vi "FaulhaberV3-Ascii_V1.vi"() -> (1 "searchnames":string[](array[string]), 2 "ID":u32[](array[numeric]), 3 "Faulhaber Objects":T3(array[cluster]))   [LabVIEW 2011] (continued)
\t<CANopenSubObject subIndex=\"0E\" name=\"Motor NTC offset\" objectType=\"7\" dataType=\"0003\" lowLimit=\"0xFFFF8000\" accessType=\"ro\" PDOmapping=\"no\" objFlags=\"00030000\" />\n\t\t\t\t\t</CANopenObject>\n\t\t\t\t\t<CANopenObject index=\"2501\" name=\"Hall scaling\" objectType=\"9\" subNumber=\"15\">\n\t\t\t\t\t\t<CANopenSubObject subIndex=\"00\" name=\"Number of entries\" objectType=\"7\" dataType=\"0005\" accessType=\"ro\" defaultValue=\"14\" PDOmapping=\"no\" />\n\t\t\t\t\t\t<CANopenSubObject subIndex=\"01\" name=\"Gain A\" objectType=\"7\" dataType=\"0006\" accessType=\"ro\" PDOmapping=\"no\" objFlags=\"00030000\" />\n\t\t\t\t\t\t<CANopenSubObject subIndex=\"02\" name=\"Hall A  offset\" objectType=\"7\" dataType=\"0006\" accessType=\"ro\" PDOmapping=\"no\" objFlags=\"00030000\" />\n\t\t\t\t\t\t<CANopenSubObject subIndex=\"03\" name=\"Hall A sin\" objectType=\"7\" dataType=\"0006\" accessType=\"ro\" PDOmapping=\"no\" objFlags=\"00030000\" />\n\t\t\t\t\t\t<CANopenSubObject subIndex=\"04\" name=\"Hall A cos\" objectType=\"7\" dataType=\"0006\" accessType=\"ro\" PDOmapping=\"no\" objFlags=\"00030000\" />\n\t\t\t\t\t\t<CANopenSubObject subIndex=\"05\" name=\"Corr A\" objectType=\"7\" dataType=\"0006\" accessType=\"ro\" PDOmapping=\"no\" objFlags=\"00030000\" />\n\t\t\t\t\t\t<CANopenSubObject subIndex=\"06\" name=\"Hall B offset\" objectType=\"7\" dataType=\"0006\" accessType=\"ro\" PDOmapping=\"no\" objFlags=\"00030000\" />\n\t\t\t\t\t\t<CANopenSubObject subIndex=\"07\" name=\"Hall B sin\" objectType=\"7\" dataType=\"0006\" accessType=\"ro\" PDOmapping=\"no\" objFlags=\"00030000\" />\n\t\t\t\t\t\t<CANopenSubObject subIndex=\"08\" name=\"Hall B cos\" objectType=\"7\" dataType=\"0006\" accessType=\"ro\" PDOmapping=\"no\" objFlags=\"00030000\" />\n\t\t\t\t\t\t<CANopenSubObject subIndex=\"09\" name=\"Corr B\" objectType=\"7\" dataType=\"0006\" accessType=\"ro\" PDOmapping=\"no\" objFlags=\"00030000\" />\n\t\t\t\t\t\t<CANopenSubObject subIndex=\"0A\" name=\"Hall C offset\" objectType=\"7\" dataType=\"0006\" accessType=\"ro\" PDOmapping=\"no\" objFlags=\"00030000\" />\n\t\t\t\t\t\t<CANopenSubObject subIndex=\"0B\" name=\"Hall C sin\" objectType=\"7\" dataType=\"0006\" accessType=\"ro\" PDOmapping=\"no\" objFlags=\"00030000\" />\n\t\t\t\t\t\t<CANopenSubObject subIndex=\"0C\" name=\"Hall C cos\" objectType=\"7\" dataType=\"0006\" accessType=\"ro\" PDOmapping=\"no\" objFlags=\"00030000\" />\n\t\t\t\t\t\t<CANopenSubObject subIndex=\"0D\" name=\"Offset A\" objectType=\"7\" dataType=\"0006\" accessType=\"ro\" PDOmapping=\"no\" objFlags=\"00030000\" />\n\t\t\t\t\t\t<CANopenSubObject subIndex=\"0E\" name=\"Offset B\" objectType=\"7\" dataType=\"0006\" accessType=\"ro\" PDOmapping=\"no\" objFlags=\"00030000\" />\n\t\t\t\t\t</CANopenObject>\n\t\t\t\t\t<CANopenObject index=\"2502\" name=\"Internal filter parameters\" objectType=\"9\" subNumber=\"14\">\n\t\t\t\t\t\t<CANopenSubObject subIndex=\"00\" name=\"Number of entries\" objectType=\"7\" dataType=\"0005\" accessType=\"ro\" defaultValue=\"13\" PDOmapping=\"no\" />\n\t\t\t\t\t\t<CANopenSubObject subIndex=\"01\" name=\"Filter time actual velocity\" objectType=\"7\" dataType=\"0006\" lowLimit=\"0\" highLimit=\"65535\" accessType=\"rw\" defaultValue=\"256\" PDOmapping=\"no\" objFlags=\"00020000\" />\n\t\t\t\t\t\t<CANopenSubObject subIndex=\"02\" name=\"Filter time IA \" objectType=\"7\" dataType=\"0006\" accessType=\"ro\" PDOmapping=\"no\" objFlags=\"00030000\" />\n\t\t\t\t\t\t<CANopenSubObject subIndex=\"03\" name=\"Filter time IB\" objectType=\"7\" dataType=\"0006\" accessType=\"ro\" PDOmapping=\"no\" objFlags=\"00030000\" />\n\t\t\t\t\t\t<CANopenSubObject subIndex=\"04\" name=\"Filter time IC\" objectType=\"7\" dataType=\"0006\" accessType=\"ro\" PDOmapping=\"no\" objFlags=\"00030000\" />\n\t\t\t\t\t\t<CANopenSubObject subIndex=\"05\" name=\"Filter time Uel\" objectType=\"7\" dataType=\"0006\" accessType=\"ro\" PDOmapping=\"no\" objFlags=\"00030000\" />\n\t\t\t\t\t\t<CANopenSubObject subIndex=\"06\" name=\"Filter time Umot\" objectType=\"7\" dataType=\"0006\" accessType=\"ro\" PDOmapping=\"no\" objFlags=\"00030000\" />\n\t\t\t\t\t\t<CANopenSubObject subIndex=\"07\" name=\"Additional filter time Uel\" objectType=\"7\" dataType=\"0006\" lowLimit=\"0x0\" accessType=\"ro\" PDOmapping=\"no\" objFlags=\"00030000\" />\n\t\t\t\t\t\t<CANopenSubObject subIndex=\"08\" name=\"Additional filter time Umot\" objectType=\"7\" dataType=\"0006\" lowLimit=\"0x0\" accessType=\"ro\" PDOmapping=\"no\" objFlags=\"00030000\" />\n\t\t\t\t\t\t<CANopenSubObject subIndex=\"09\" name=\"Filter time Iq thermal model\" objectType=\"7\" dataType=\"0006\" accessType=\"ro\" PDOmapping=\"no\" objFlags=\"00030000\" />\n\t\t\t\t\t\t<CANopenSubObject subIndex=\"0A\" name=\"Filter time Id thermal model\" objectType=\"7\" dataType=\"0006\" accessType=\"ro\" PDOmapping=\"no\" objFlags=\"00030000\" />\n\t\t\t\t\t\t<CANopenSubObject subIndex=\"0B\" name=\"Filter time Imot thermal model\" objectType=\"7\" dataType=\"0006\" accessType=\"ro\" PDOmapping=\"no\" objFlags=\"00030000\" />\n\t\t\t\t\t\t<CANopenSubObject subIndex=\"0C\" name=\"Filter time setpoint voltage model\" objectType=\"7\" dataType=\"0006\" accessType=\"ro\" PDOmapping=\"no\" objFlags=\"00030000\" />\n\t\t\t\t\t\t<CANopenSubObject subIndex=\"0D\" name=\"Filter time electrical time constant\" objectType=\"7\" dataType=\"0006\" lowLimit=\"0\" highLimit=\"65535\" accessType=\"rw\" PDOmapping=\"no\" objFlags=\"00020000\" />\n\t\t\t\t\t</CANopenObject>\n\t\t\t\t\t<CANopenObject index=\"2503\" name=\"Boot options\" objectType=\"7\" dataType=\"0006\" lowLimit=\"0\" highLimit=\"2\" accessType=\"rw\" defaultValue=\"1\" PDOmapping=\"no\" objFlags=\"00020000\" />\n\t\t\t\t\t<CANopenObject index=\"2504\" name=\"Hall compensation\" objectType=\"9\" subNumber=\"13\">\n\t\t\t\t\t\t<CANopenSubObject subIndex=\"00\" name=\"Number of entries\" objectType=\"7\" dataType=\"0005\" accessType=\"ro\" defaultValue=\"12\" PDOmapping=\"no\" />\n\t\t\t\t\t\t<CANopenSubObject subIndex=\"01\" name=\"Entry 01\" objectType=\"7\" dataType=\"0003\" accessType=\"ro\" PDOmapping=\"no\" objFlags=\"00030000\" />\n\t\t\t\t\t\t<CANopenSubObject subIndex=\"02\" name=\"Entry 02\" objectType=\"7\" dataType=\"0003\" accessType=\"ro\" PDOmapping=\"no\" objFlags=\"00030000\" />\n\t\t\t\t\t\t<CANopenSubObject subIndex=\"03\" name=\"Entry 03\" objectType=\"7\" dataType=\"0003\" accessType=\"ro\" PDOmapping=\"no\" objFlags=\"00030000\" />\n\t\t\t\t\t\t<CANopenSubObject subIndex=\"04\" name=\"Entry 04\" objectType=\"7\" dataType=\"0003\" accessType=\"ro\" PDOmapping=\"no\" objFlags=\"00030000\" />\n\t\t\t\t\t\t<CANopenSubObject subIndex=\"05\" name=\"Entry 05\" objectType=\"7\" dataType=\"0003\" accessType=\"ro\" PDOmapping=\"no\" objFlags=\"00030000\" />\n\t\t\t\t\t\t<CANopenSubObject subIndex=\"06\" name=\"Entry 06\" objectType=\"7\" dataType=\"0003\" accessType=\"ro\" PDOmapping=\"no\" objFlags=\"00030000\" />\n\t\t\t\t\t\t<CANopenSubObject subIndex=\"07\" name=\"Entry 07\" objectType=\"7\" dataType=\"0003\" accessType=\"ro\" PDOmapping=\"no\" objFlags=\"00030000\" />\n\t\t\t\t\t\t<CANopenSubObject subIndex=\"08\" name=\"Entry 08\" objectType=\"7\" dataType=\"0003\" accessType=\"ro\" PDOmapping=\"no\" objFlags=\"00030000\" />\n\t\t\t\t\t\t<CANopenSubObject subIndex=\"09\" name=\"Entry 09\" objectType=\"7\" dataType=\"0003\" accessType=\"ro\" PDOmapping=\"no\" objFlags=\"00030000\" />\n\t\t\t\t\t\t<CANopenSubObject subIndex=\"0A\" name=\"Entry 10\" objectType=\"7\" dataType=\"0003\" accessType=\"ro\" PDOmapping=\"no\" objFlags=\"00030000\" />\n\t\t\t\t\t\t<CANopenSubObject subIndex=\"0B\" name=\"Entry 11\" objectType=\"7\" dataType=\"0003\" accessType=\"ro\" PDOmapping=\"no\" objFlags=\"00030000\" />\n\t\t\t\t\t\t<CANopenSubObject subIndex=\"0C\" name=\"Entry 12\" objectType=\"7\" dataType=\"0003\" accessType=\"ro\" PDOmapping=\"no\" objFlags=\"00030000\" />\n\t\t\t\t\t</CANopenObject>\n\t\t\t\t\t<CANopenObject index=\"2506\" name=\"Encoder compensation\" objectType=\"9\" subNumber=\"65\">\n\t\t\t\t\t\t<CANopenSubObject subIndex=\"00\" name=\"Number of entries\" objectType=\"7\" dataType=\"0005\" accessType=\"ro\" defaultValue=\"64\" PDOmapping=\"no\" />\n\t\t\t\t\t\t<CANopenSubObject subIndex=\"01\" name=\"Value 0\" objectType=\"7\" dataType=\"0003\" lowLimit=\"-32768\" highLimit=\"32767\" accessType=\"rw\" defaultValue=\"0\" PDOmapping=\"no\" objFlags=\"00020000\" />\n\t\t\t\t\t\t<CANopenSubObject subIndex=\"02\" name=\"Value 1\" objectType=\"7\" dataType=\"0003\" lowLimit=\"-32768\" highLimit=\"32767\" accessType=\"rw\" defaultValue=\"0\" PDOmapping=\"no\" objFlags=\"00020000\" />\n\t\t\t\t\t\t<CANopenSubObject subIndex=\"03\" name=\"Value 2\" objectType=\"7\" dataType=\"0003\" lowLimit=\"-32768\" highLimit=\"32767\" accessType=\"rw\" defaultValue=\"0\" PDOmapping=\"no\" objFlags=\"00020000\" />\n\t\t\t\t\t\t<CANopenSubObject subIndex=\"04\" name=\"Value 3\" objectType=\"7\" dataType=\"0003\" lowLimit=\"-32768\" highLimit=\"32767\" accessType=\"rw\" defaultValue=\"0\" PDOmapping=\"no\" objFlags=\"00020000\" />\n\t\t\t\t\t\t<CANopenSubObject subIndex=\"05\" name=\"Value 4\" objectType=\"7\" dataType=\"0003\" lowLimit=\"-32768\" highLimit=\"32767\" accessType=\"rw\" defaultValue=\"0\" PDOmapping=\"no\" objFlags=\"00020000\" />\n\t\t\t\t\t\t<CANopenSubObject subIndex=\"06\" name=\"Value 5\" objectType=\"7\" dataType=\"0003\" lowLimit=\"-32768\" highLimit=\"32767\" accessType=\"rw\" defaultValue=\"0\" PDOmapping=\"no\" objFlags=\"00020000\" />\n\t\t\t\t\t\t<CANopenSubObject subIndex=\"07\" name=\"Value 6\" objectType=\"7\" dataType=\"0003\" lowLimit=\"-32768\" highLimit=\"32767\" accessType=\"rw\" defaultValue=\"0\" PDOmapping=\"no\" objFlags=\"00020000\" />\n\t\t\t\t\t\t<CANopenSubObject subIndex=\"08\" name=\"Value 7\" objectType=\"7\" dataType=\"0003\" lowLimit=\"-32768\" highLimit=\"32767\" accessType=\"rw\" defaultValue=\"0\" PDOmapping=\"no\" objFlags=\"00020000\" />\n\t\t\t\t\t\t<CANopenSubObject subIndex=\"09\" name=\"Value 8\" objectType=\"7\" dataType=\"0003\" lowLimit=\"-32768\" highLimit=\"32767\" accessType=\"rw\" defaultValue=\"0\" PDOmapping=\"no\" objFlags=\"00020000\" />\n\t\t\t\t\t\t<CANopenSubObject subIndex=\"0A\" name=\"Value 9\" objectType=\"7\" dataType=\"0003\" lowLimit=\"-32768\" highLimit=\"32767\" accessType=\"rw\" defaultValue=\"0\" PDOmapping=\"no\" objFlags=\"00020000\" />\n\t\t\t\t\t\t<CANopenSubObject subIndex=\"0B\" name=\"Value 10\" objectType=\"7\" dataType=\"0003\" lowLimit=\"-32768\" highLimit=\"32767\" accessType=\"rw\" defaultValue=\"0\" PDOmapping=\"no\" objFlags=\"00020000\" />\n\t\t\t\t\t\t<CANopenSubObject subIndex=\"0C\" name=\"Value 11\" objectType=\"7\" dataType=\"0003\" lowLimit=\"-32768\" highLimit=\"32767\" accessType=\"rw\" defaultValue=\"0\" PDOmapping=\"no\" objFlags=\"00020000\" />\n\t\t\t\t\t\t<CANopenSubObject subIndex=\"0D\" name=\"Value 12\" objectType=\"7\" dataType=\"0003\" lowLimit=\"-32768\" highLimit=\"32767\" accessType=\"rw\" defaultValue=\"0\" PDOmapping=\"no\" objFlags=\"00020000\" />\n\t\t\t\t\t\t<CANopenSubObject subIndex=\"0E\" name=\"Value 13\" objectType=\"7\" dataType=\"0003\" lowLimit=\"-32768\" highLimit=\"32767\" accessType=\"rw\" defaultValue=\"0\" PDOmapping=\"no\" objFlags=\"00020000\" />\n\t\t\t\t\t\t<CANopenSubObject subIndex=\"0F\" name=\"Value 14\" objectType=\"7\" dataType=\"0003\" lowLimit=\"-32768\" highLimit=\"32767\" accessType=\"rw\" defaultValue=\"0\" PDOmapping=\"no\" objFlags=\"00020000\" />\n\t\t\t\t\t\t<CANopenSubObject subIndex=\"10\" name=\"Value 15\" objectType=\"7\" dataType=\"0003\" lowLimit=\"-32768\" highLimit=\"32767\" accessType=\"rw\" defaultValue=\"0\" PDOmapping=\"no\" objFlags=\"00020000\" />\n\t\t\t\t\t\t<CANopenSubObject subIndex=\"11\" name=\"Value 16\" objectType=\"7\" dataType=\"0003\" lowLimit=\"-32768\" highLimit=\"32767\" accessType=\"rw\" defaultValue=\"0\" PDOmapping=\"no\" objFlags=\"00020000\" />\n\t\t\t\t\t\t<CANopenSubObject subIndex=\"12\" name=\"Value 17\" objectType=\"7\" dataType=\"0003\" lowLimit=\"-32768\" highLimit=\"32767\" accessType=\"rw\" defaultValue=\"0\" PDOmapping=\"no\" objFlags=\"00020000\" />\n\t\t\t\t\t\t<CANopenSubObject subIndex=\"13\" name=\"Value 18\" objectType=\"7\" dataType=\"0003\" lowLimit=\"-32768\" highLimit=\"32767\" accessType=\"rw\" defaultValue=\"0\" PDOmapping=\"no\" objFlags=\"00020000\" />\n\t\t\t\t\t\t<CANopenSubObject subIndex=\"14\" name=\"Value 19\" objectType=\"7\" dataType=\"0003\" lowLimit=\"-32768\" highLimit=\"32767\" accessType=\"rw\" defaultValue=\"0\" PDOmapping=\"no\" objFlags=\"00020000\" />\n\t\t\t\t\t\t<CANopenSubObject subIndex=\"15\" name=\"Value 20\" objectType=\"7\" dataType=\"0003\" lowLimit=\"-32768\" highLimit=\"32767\" accessType=\"rw\" defaultValue=\"0\" PDOmapping=\"no\" objFlags=\"00020000\" />\n\t\t\t\t\t\t<CANopenSubObject subIndex=\"16\" name=\"Value 21\" objectType=\"7\" dataType=\"0003\" lowLimit=\"-32768\" highLimit=\"32767\" accessType=\"rw\" defaultValue=\"0\" PDOmapping=\"no\" objFlags=\"00020000\" />\n\t\t\t\t\t\t<CANopenSubObject subIndex=\"17\" name=\"Value 22\" objectType=\"7\" dataType=\"0003\" lowLimit=\"-32768\" highLimit=\"32767\" accessType=\"rw\" defaultValue=\"0\" PDOmapping=\"no\" objFlags=\"00020000\" />\n\t\t\t\t\t\t<CANopenSubObject subIndex=\"18\" name=\"Value 23\" objectType=\"7\" dataType=\"0003\" lowLimit=\"-32768\" highLimit=\"32767\" accessType=\"rw\" defaultValue=\"0\" PDOmapping=\"no\" objFlags=\"00020000\" />\n\t\t\t\t\t\t<CANopenSubObject subIndex=\"19\" name=\"Value 24\" objectType=\"7\" dataType=\"0003\" lowLimit=\"-32768\" highLimit=\"32767\" accessType=\"rw\" defaultValue=\"0\" PDOmapping=\"no\" objFlags=\"00020000\" />\n\t\t\t\t\t\t<CANopenSubObject subIndex=\"1A\" name=\"Value 25\" objectType=\"7\" dataType=\"0003\" lowLimit=\"-32768\" highLimit=\"32767\" accessType=\"rw\" defaultValue=\"0\" PDOmapping=\"no\" objFlags=\"00020000\" />\n\t\t\t\t\t\t<CANopenSubObject subIndex=\"1B\" name=\"Value 26\" objectType=\"7\" dataType=\"0003\" lowLimit=\"-32768\" highLimit=\"32767\" accessType=\"rw\" defaultValue=\"0\" PDOmapping=\"no\" objFlags=\"00020000\" />\n\t\t\t\t\t\t<CANopenSubObject subIndex=\"1C\" name=\"Value 27\" objectType=\"7\" dataType=\"0003\" lowLimit=\"-32768\" highLimit=\"32767\" accessType=\"rw\" defaultValue=\"0\" PDOmapping=\"no\" objFlags=\"00020000\" />\n\t\t\t\t\t\t<CANopenSubObject subIndex=\"1D\" name=\"Value 28\" objectType=\"7\" dataType=\"0003\" lowLimit=\"-32768\" highLimit=\"32767\" accessType=\"rw\" defaultValue=\"0\" PDOmapping=\"no\" objFlags=\"00020000\" />\n\t\t\t\t\t\t<CANopenSubObject subIndex=\"1E\" name=\"Value 29\" objectType=\"7\" dataType=\"0003\" lowLimit=\"-32768\" highLimit=\"32767\" accessType=\"rw\" defaultValue=\"0\" PDOmapping=\"no\" objFlags=\"00020000\" />\n\t\t\t\t\t\t<CANopenSubObject subIndex=\"1F\" name=\"Value 30\" objectType=\"7\" dataType=\"0003\" lowLimit=\"-32768\" highLimit=\"32767\" accessType=\"rw\" defaultValue=\"0\" PDOmapping=\"no\" objFlags=\"00020000\" />\n\t\t\t\t\t\t<CANopenSubObject subIndex=\"20\" name=\"Value 31\" objectType=\"7\" dataType=\"0003\" lowLimit=\"-32768\" highLimit=\"32767\" accessType=\"rw\" defaultValue=\"0\" PDOmapping=\"no\" objFlags=\"00020000\" />\n\t\t\t\t\t\t<CANopenSubObject subIndex=\"21\" name=\"Value 32\" objectType=\"7\" dataType=\"0003\" lowLimit=\"-32768\" highLimit=\"32767\" accessType=\"rw\" defaultValue=\"0\" PDOmapping=\"no\" objFlags=\"00020000\" />\n\t\t\t\t\t\t<CANopenSubObject subIndex=\"22\" name=\"Value 33\" objectType=\"7\" dataType=\"0003\" lowLimit=\"-32768\" highLimit=\"32767\" accessType=\"rw\" defaultValue=\"0\" PDOmapping=\"no\" objFlags=\"00020000\" />\n\t\t\t\t\t\t<CANopenSubObject subIndex=\"23\" name=\"Value 34\" objectType=\"7\" dataType=\"0003\" lowLimit=\"-32768\" highLimit=\"32767\" accessType=\"rw\" defaultValue=\"0\" PDOmapping=\"no\" objFlags=\"00020000\" />\n\t\t\t\t\t\t<CANopenSubObject subIndex=\"24\" name=\"Value 35\" objectType=\"7\" dataType=\"0003\" lowLimit=\"-32768\" highLimit=\"32767\" accessType=\"rw\" defaultValue=\"0\" PDOmapping=\"no\" objFlags=\"00020000\" />\n\t\t\t\t\t\t<CANopenSubObject subIndex=\"25\" name=\"Value 36\" objectType=\"7\" dataType=\"0003\" lowLimit=\"-32768\" highLimit=\"32767\" accessType=\"rw\" defaultValue=\"0\" PDOmapping=\"no\" objFlags=\"00020000\" />\n\t\t\t\t\t\t<CANopenSubObject subIndex=\"26\" name=\"Value 37\" objectType=\"7\" dataType=\"0003\" lowLimit=\"-32768\" highLimit=\"32767\" accessType=\"rw\" defaultValue=\"0\" PDOmapping=\"no\" objFlags=\"00020000\" />\n\t\t\t\t\t\t<CANopenSubObject subIndex=\"27\" name=\"Value 38\" objectType=\"7\" dataType=\"0003\" lowLimit=\"-32768\" highLimit=\"32767\" accessType=\"rw\" defaultValue=\"0\" PDOmapping=\"no\" objFlags=\"00020000\" />\n\t\t\t\t\t\t<CANopenSubObject subIndex=\"28\" name=\"Value 39\" objectType=\"7\" dataType=\"0003\" lowLimit=\"-32768\" highLimit=\"32767\" accessType=\"rw\" defaultValue=\"0\" PDOmapping=\"no\" objFlags=\"00020000\" />\n\t\t\t\t\t\t<CANopenSubObject subIndex=\"29\" name=\"Value 40\" objectType=\"7\" dataType=\"0003\" lowLimit=\"-32768\" highLimit=\"32767\" accessType=\"rw\" defaultValue=\"0\" PDOmapping=\"no\" objFlags=\"00020000\" />\n\t\t\t\t\t\t<CANopenSubObject subIndex=\"2A\" name=\"Value 41\" objectType=\"7\" dataType=\"0003\" lowLimit=\"-32768\" highLimit=\"32767\" accessType=\"rw\" defaultValue=\"0\" PDOmapping=\"no\" objFlags=\"00020000\" />\n\t\t\t\t\t\t<CANopenSubObject subIndex=\"2B\" name=\"Value 42\" objectType=\"7\" dataType=\"0003\" lowLimit=\"-32768\" highLimit=\"32767\" accessType=\"rw\" defaultValue=\"0\" PDOmapping=\"no\" objFlags=\"00020000\" />\n\t\t\t\t\t\t<CANopenSubObject subIndex=\"2C\" name=\"Value 43\" objectType=\"7\" dataType=\"0003\" lowLimit=\"-32768\" highLimit=\"32767\" accessType=\"rw\" defaultValue=\"0\" PDOmapping=\"no\" objFlags=\"00020000\" />\n\t\t\t\t\t\t<CANopenSubObject subIndex=\"2D\" name=\"Value 44\" objectType=\"7\" dataType=\"0003\" lowLimit=\"-32768\" highLimit=\"32767\" accessType=\"rw\" defaultValue=\"0\" PDOmapping=\"no\" objFlags=\"00020000\" />\n\t\t\t\t\t\t<CANopenSubObject subIndex=\"2E\" name=\"Value 45\" objectType=\"7\" dataType=\"0003\" lowLimit=\"-32768\" highLimit=\"32767\" accessType=\"rw\" defaultValue=\"0\" PDOmapping=\"no\" objFlags=\"00020000\" />\n\t\t\t\t\t\t<CANopenSubObject subIndex=\"2F\" name=\"Value 46\" objectType=\"7\" dataType=\"0003\" lowLimit=\"-32768\" highLimit=\"32767\" accessType=\"rw\" defaultValue=\"0\" PDOmapping=\"no\" objFlags=\"00020000\" />\n\t\t\t\t\t\t<CANopenSubObject subIndex=\"30\" name=\"Value 47\" objectType=\"7\" dataType=\"0003\" lowLimit=\"-32768\" highLimit=\"32767\" accessType=\"rw\" defaultValue=\"0\" PDOmapping=\"no\" objFlags=\"00020000\" />\n\t\t\t\t\t\t<CANopenSubObject subIndex=\"31\" name=\"Value 48\" objectType=\"7\" dataType=\"0003\" lowLimit=\"-32768\" highLimit=\"32767\" accessType=\"rw\" defaultValue=\"0\" PDOmapping=\"no\" objFlags=\"00020000\" />\n\t\t\t\t\t\t<CANopenSubObject subIndex=\"32\" name=\"Value 49\" objectType=\"7\" dataType=\"0003\" lowLimit=\"-32768\" highLimit=\"32767\" accessType=\"rw\" defaultValue=\"0\" PDOmapping=\"no\" objFlags=\"00020000\" />\n\t\t\t\t\t\t<CANopenSubObject subIndex=\"33\" name=\"Value 50\" objectType=\"7\" dataType=\"0003\" lowLimit=\"-32768\" highLimit=\"32767\" accessType=\"rw\" defaultValue=\"0\" PDOmapping=\"no\" objFlags=\"00020000\" />\n\t\t\t\t\t\t<CANopenSubObject subIndex=\"34\" name=\"Value 51\" objectType=\"7\" dataType=\"0003\" lowLimit=\"-32768\" highLimit=\"32767\" accessType=\"rw\" defaultValue=\"0\" PDOmapping=\"no\" objFlags=\"00020000\" />\n\t\t\t\t\t\t<CANopenSubObject subIndex=\"35\" name=\"Value 52\" objectType=\"7\" dataType=\"0003\" lowLimit=\"-32768\" highLimit=\"32767\" accessType=\"rw\" defaultValue=\"0\" PDOmapping=\"no\" objFlags=\"00020000\" />\n\t\t\t\t\t\t<CANopenSubObject subIndex=\"36\" name=\"Value 53\" objectType=\"7\" dataType=\"0003\" lowLimit=\"-32768\" highLimit=\"32767\" accessType=\"rw\" defaultValue=\"0\" PDOmapping=\"no\" objFlags=\"00020000\" />\n\t\t\t\t\t\t<CANopenSubObject subIndex=\"37\" name=\"Value 54\" objectType=\"7\" dataType=\"0003\" lowLimit=\"-32768\" highLimit=\"32767\" accessType=\"rw\" defaultValue=\"0\" PDOmapping=\"no\" objFlags=\"00020000\" />\n\t\t\t\t\t\t<CANopenSubObject subIndex=\"38\" name=\"Value 55\" objectType=\"7\" dataType=\"0003\" lowLimit=\"-32768\" highLimit=\"32767\" accessType=\"rw\" defaultValue=\"0\" PDOmapping=\"no\" objFlags=\"00020000\" />\n\t\t\t\t\t\t<CANopenSubObject subIndex=\"39\" name=\"Value 56\" objectType=\"7\" dataType=\"0003\" lowLimit=\"-32768\" highLimit=\"32767\" accessType=\"rw\" defaultValue=\"0\" PDOmapping=\"no\" objFlags=\"00020000\" />\n\t\t\t\t\t\t<CANopenSubObject subIndex=\"3A\" name=\"Value 57\" objectType=\"7\" dataType=\"0003\" lowLimit=\"-32768\" highLimit=\"32767\" accessType=\"rw\" defaultValue=\"0\" PDOmapping=\"no\" objFlags=\"00020000\" />\n\t\t\t\t\t\t<CANopenSubObject subIndex=\"3B\" name=\"Value 58\" objectType=\"7\" dataType=\"0003\" lowLimit=\"-32768\" highLimit=\"32767\" accessType=\"rw\" defaultValue=\"0\" PDOmapping=\"no\" objFlags=\"00020000\" />\n\t\t\t\t\t\t<CANopenSubObject subIndex=\"3C\" name=\"Value 59\" objectType=\"7\" dataType=\"0003\" lowLimit=\"-32768\" highLimit=\"32767\" accessType=\"rw\" defaultValue=\"0\" PDOmapping=\"no\" objFlags=\"00020000\" />\n\t\t\t\t\t\t<CANopenSubObject subIndex=\"3D\" name=\"Value 60\" objectType=\"7\" dataType=\"0003\" lowLimit=\"-32768\" highLimit=\"32767\" accessType=\"rw\" defaultValue=\"0\" PDOmapping=\"no\" objFlags=\"00020000\" />\n\t\t\t\t\t\t<CANopenSubObject subIndex=\"3E\" name=\"Value 61\" objectType=\"7\" dataType=\"0003\" lowLimit=\"-32768\" highLimit=\"32767\" accessType=\"rw\" defaultValue=\"0\" PDOmapping=\"no\" objFlags=\"00020000\" />\n\t\t\t\t\t\t<CANopenSubObject subIndex=\"3F\" name=\"Value 62\" objectType=\"7\" dataType=\"0003\" lowLimit=\"-32768\" highLimit=\"32767\" accessType=\"rw\" defaultValue=\"0\" PDOmapping=\"no\" objFlags=\"00020000\" />\n\t\t\t\t\t\t<CANopenSubObject subIndex=\"40\" name=\"Value 63\" objectType=\"7\" dataType=\"0003\" lowLimit=\"-32768\" highLimit=\"32767\" accessType=\"rw\" defaultValue=\"0\" PDOmapping=\"no\" objFlags=\"00020000\" />\n\t\t\t\t\t</CANopenObject>\n\t\t\t\t\t<CANopenObject index=\"250A\" name=\"Pwm frequency\" objectType=\"7\" dataType=\"0005\" lowLimit=\"1\" highLimit=\"10\" accessType=\"rw\" defaultValue=\"4\" PDOmapping=\"no\" objFlags=\"00020000\" />\n\t\t\t\t\t<CANopenObject index=\"250F\" name=\"250F_00\" objectType=\"7\" dataType=\"0005\" lowLimit=\"0\" highLimit=\"255\" accessType=\"wo\" defaultValue=\"0\" PDOmapping=\"no\" objFlags=\"00020003\" />\n\t\t\t\t\t<CANopenObject index=\"2600\" name=\"Drive system gear\" objectType=\"9\" subNumber=\"3\">\n\t\t\t\t\t\t<CANopenSubObject subIndex=\"00\" name=\"Number of entries\" objectType=\"7\" dataType=\"0005\" accessType=\"ro\" defaultValue=\"2\" PDOmapping=\"no\" />\n\t\t\t\t\t\t<CANopenSubObject subIndex=\"01\" name=\"Gear ratio num\" objectType=\"7\" dataType=\"0007\" lowLimit=\"1\" highLimit=\"4294967295\" accessType=\"rw\" defaultValue=\"1\" PDOmapping=\"no\" objFlags=\"00020000\" />\n\t\t\t\t\t\t<CANopenSubObject subIndex=\"02\" name=\"Gear ratio den\" objectType=\"7\" dataType=\"0007\" lowLimit=\"1\" highLimit=\"4294967295\" accessType=\"rw\" defaultValue=\"1\" PDOmapping=\"no\" objFlags=\"00020000\" />\n\t\t\t\t\t</CANopenObject>\n\t\t\t\t\t<CANopenObject index=\"2601\" name=\"Drive system load transmission\" objectType=\"9\" subNumber=\"4\">\n\t\t\t\t\t\t<CANopenSubObject subIndex=\"00\" name=\"Number of entries\" objectType=\"7\" dataType=\"0005\" accessType=\"ro\" defaultValue=\"3\" PDOmapping=\"no\" />\n\t\t\t\t\t\t<CANopenSubObject subIndex=\"01\" name=\"Load transmission\" objectType=\"7\" dataType=\"0005\" lowLimit=\"0\" highLimit=\"255\" accessType=\"rw\" PDOmapping=\"no\" objFlags=\"00020000\" />\n\t\t\t\t\t\t<CANopenSubObject subIndex=\"02\" name=\"Load transmission ratio num\" objectType=\"7\" dataType=\"0007\" lowLimit=\"1\" highLimit=\"4294967295\" accessType=\"rw\" defaultValue=\"1\" PDOmapping=\"no\" objFlags=\"00020000\" />\n\t\t\t\t\t\t<CANopenSubObject subIndex=\"03\" name=\"Load transmission ratio den\" objectType=\"7\" dataType=\"0007\" lowLimit=\"1\" highLimit=\"4294967295\" accessType=\"rw\" defaultValue=\"1\" PDOmapping=\"no\" objFlags=\"00020000\" />\n\t\t\t\t\t</CANopenObject>\n\t\t\t\t\t<CANopenObject index=\"2602\" name=\"Drive system numbers\" objectType=\"9\" subNumber=\"4\">\n\t\t\t\t\t\t<CANopenSubObject subIndex=\"00\" name=\"Number of entries\" objectType=\"7\" dataType=\"0005\" accessType=\"ro\" defaultValue=\"3\" PDOmapping=\"no\" />\n\t\t\t\t\t\t<CANopenSubObject subIndex=\"01\" name=\"Gear catalog number\" objectType=\"7\" dataType=\"0009\" accessType=\"rw\" defaultValue=\"0\" PDOmapping=\"no\" objFlags=\"00020000\" />\n\t\t\t\t\t\t<CANopenSubObject subIndex=\"02\" name=\"Encoder cataloge number\" objectType=\"7\" dataType=\"0009\" accessType=\"rw\" defaultValue=\"0\" PDOmapping=\"no\" objFlags=\"00020000\" />\n\t\t\t\t\t\t<CANopenSubObject subIndex=\"03\" name=\"Drive combination number\" objectType=\"7\" dataType=\"0009\" accessType=\"rw\" defaultValue=\"0\" PDOmapping=\"no\" objFlags=\"00020000\" />\n\t\t\t\t\t</CANopenObject>\n\t\t\t\t\t<CANopenObject index=\"2603\" name=\"Drive system units\" objectType=\"9\" subNumber=\"3\">\n\t\t\t\t\t\t<CANopenSubObject subIndex=\"00\" name=\"Number of entries\" objectType=\"7\" dataType=\"0005\" accessType=\"ro\" defaultValue=\"2\" PDOmapping=\"no\" />\n\t\t\t\t\t\t<CANopenSubObject subIndex=\"01\" name=\"Unit reference\" objectType=\"7\" dataType=\"0005\" lowLimit=\"0\" highLimit=\"255\" accessType=\"rw\" defaultValue=\"0\" PDOmapping=\"no\" objFlags=\"00020000\" />\n\t\t\t\t\t\t<CANopenSubObject subIndex=\"02\" name=\"Unit names\" objectType=\"7\" dataType=\"0009\" accessType=\"rw\" defaultValue=\"0\" PDOmapping=\"no\" objFlags=\"00020000\" />\n\t\t\t\t\t</CANopenObject>\n\t\t\t\t\t<CANopenObject index=\"2604\" name=\"Nominal voltage\" objectType=\"7\" dataType=\"0006\" lowLimit=\"0\" highLimit=\"65535\" accessType=\"rw\" PDOmapping=\"no\" objFlags=\"00020000\" />\n\t\t\t\t\t<CANopenObject index=\"2605\" name=\"Drive system settings\" objectType=\"7\" dataType=\"0007\" lowLimit=\"0\" highLimit=\"4294967295\" accessType=\"rw\" PDOmapping=\"no\" objFlags=\"00020000\" />\n\t\t\t\t\t<CANopenObject index=\"2610\" name=\"OEM DeviceData\" objectType=\"9\" subNumber=\"4\">\n\t\t\t\t\t\t<CANopenSubObject subIndex=\"00\" name=\"Number of entries\" objectType=\"7\" dataType=\"0005\" accessType=\"ro\" defaultValue=\"3\" PDOmapping=\"no\" />\n\t\t\t\t\t\t<CANopenSubObject subIndex=\"01\" name=\"OEM product descriptor \" objectType=\"7\" dataType=\"0009\" accessType=\"rw\" defaultValue=\"0\" PDOmapping=\"no\" objFlags=\"00020000\" />\n\t\t\t\t\t\t<CANopenSubObject subIndex=\"02\" name=\"OEM product code\" objectType=\"7\" dataType=\"0009\" accessType=\"rw\" defaultValue=\"0\" PDOmapping=\"no\" objFlags=\"00020000\" />\n\t\t\t\t\t\t<CANopenSubObject subIndex=\"03\" name=\"OEM serial number\" objectType=\"7\" dataType=\"0007\" lowLimit=\"0\" highLimit=\"4294967295\" accessType=\"rw\" defaultValue=\"0\" PDOmapping=\"no\" objFlags=\"00020000\" />\n\t\t\t\t\t</CANopenObject>\n\t\t\t\t\t<CANopenObject index=\"3000\" name=\"User programs\" objectType=\"8\" subNumber=\"9\">\n\t\t\t\t\t\t<CANopenSubObject subIndex=\"00\" name=\"Number of entries\" objectType=\"7\" dataType=\"0005\" accessType=\"ro\" defaultValue=\"8\" PDOmapping=\"no\" />\n\t\t\t\t\t\t<CANopenSubObject subIndex=\"01\" name=\"User program 1 start address\" objectType=\"7\" dataType=\"0006\" lowLimit=\"0\" highLimit=\"65535\" accessType=\"rw\" defaultValue=\"0xFFFF\" PDOmapping=\"no\" objFlags=\"00020001\" />\n\t\t\t\t\t\t<CANopenSubObject subIndex=\"02\" name=\"User program 2 start address\" objectType=\"7\" dataType=\"0006\" lowLimit=\"0\" highLimit=\"65535\" accessType=\"rw\" defaultValue=\"0xFFFF\" PDOmapping=\"no\" objFlags=\"00020001\" />\n\t\t\t\t\t\t<CANopenSubObject subIndex=\"03\" name=\"User program 3 start address\" objectType=\"7\" dataType=\"0006\" lowLimit=\"0\" highLimit=\"65535\" accessType=\"rw\" defaultValue=\"0xFFFF\" PDOmapping=\"no\" objFlags=\"00020001\" />\n\t\t\t\t\t\t<CANopenSubObject subIndex=\"04\" name=\"User program 4 start address\" objectType=\"7\" dataType=\"0006\" lowLimit=\"0\" highLimit=\"65535\" accessType=\"rw\" defaultValue=\"0xFFFF\" PDOmapping=\"no\" objFlags=\"00020001\" />\n\t\t\t\t\t\t<CANopenSubObject subIndex=\"05\" name=\"User program 5 start address\" objectType=\"7\" dataType=\"0006\" lowLimit=\"0\" highLimit=\"65535\" accessType=\"rw\" defaultValue=\"0xFFFF\" PDOmapping=\"no\" objFlags=\"00020001\" />\n\t\t\t\t\t\t<CANopenSubObject subIndex=\"06\" name=\"User program 6 start address\" objectType=\"7\" dataType=\"0006\" lowLimit=\"0\" highLimit=\"65535\" accessType=\"rw\" defaultValue=\"0xFFFF\" PDOmapping=\"no\" objFlags=\"00020001\" />\n\t\t\t\t\t\t<CANopenSubObject subIndex=\"07\" name=\"User program 7 start address\" objectType=\"7\" dataType=\"0006\" lowLimit=\"0\" highLimit=\"65535\" accessType=\"rw\" defaultValue=\"0xFFFF\" PDOmapping=\"no\" objFlags=\"00020001\" />\n\t\t\t\t\t\t<CANopenSubObject subIndex=\"08\" name=\"User program 8 start address\" objectType=\"7\" dataType=\"0006\" lowLimit=\"0\" highLimit=\"65535\" accessType=\"rw\" defaultValue=\"0xFFFF\" PDOmapping=\"no\" objFlags=\"00020001\" />\n\t\t\t\t\t</CANopenObject>\n\t\t\t\t\t<CANopenObject index=\"3001\" name=\"Active program\" objectType=\"9\" subNumber=\"10\">\n\t\t\t\t\t\t<CANopenSubObject subIndex=\"00\" name=\"Number of entries\" objectType=\"7\" dataType=\"0005\" accessType=\"ro\" defaultValue=\"10\" PDOmapping=\"no\" />\n\t\t\t\t\t\t<CANopenSubObject subIndex=\"01\" name=\"Actual program command\" objectType=\"7\" dataType=\"0005\" lowLimit=\"0\" highLimit=\"255\" accessType=\"rw\" defaultValue=\"0\" PDOmapping=\"no\" objFlags=\"00020001\" />\n\t\t\t\t\t\t<CANopenSubObject subIndex=\"02\" name=\"Actual program number\" objectType=\"7\" dataType=\"0005\" lowLimit=\"0\" highLimit=\"255\" accessType=\"rw\" defaultValue=\"0\" PDOmapping=\"no\" objFlags=\"00020001\" />\n\t\t\t\t\t\t<CANopenSubObject subIndex=\"03\" name=\"Actual program position\" objectType=\"7\" dataType=\"0006\" accessType=\"ro\" PDOmapping=\"no\" objFlags=\"00020000\" />\n\t\t\t\t\t\t<CANopenSubObject subIndex=\"04\" name=\"Actual program state\" objectType=\"7\" dataType=\"0005\" accessType=\"ro\" PDOmapping=\"no\" objFlags=\"00020000\" />\n\t\t\t\t\t\t<CANopenSubObject subIndex=\"05\" name=\"Breakpoint address\" objectType=\"7\" dataType=\"0006\" lowLimit=\"0\" highLimit=\"65535\" accessType=\"rw\" defaultValue=\"0xFFFF\" PDOmapping=\"no\" objFlags=\"00020001\" />\n\t\t\t\t\t\t<CANopenSubObject subIndex=\"07\" name=\"Upload/Download buffer\" objectType=\"7\" dataType=\"0009\" accessType=\"rw\" defaultValue=\"0\" PDOmapping=\"no\" objFlags=\"00020003\" />\n\t\t\t\t\t\t<CANopenSubObject subIndex=\"08\" name=\"Error state\" objectType=\"7\" dataType=\"0005\" accessType=\"ro\" PDOmapping=\"no\" objFlags=\"00020000\" />\n\t\t\t\t\t\t<CANopenSubObject subIndex=\"09\" name=\"Error code\" objectType=\"7\" dataType=\"0006\" accessType=\"ro\" PDOmapping=\"no\" objFlags=\"00020000\" />\n\t\t\t\t\t\t<CANopenSubObject subIndex=\"0A\" name=\"Program memory\" objectType=\"7\" dataType=\"0006\" accessType=\"ro\" defaultValue=\"0\" PDOmapping=\"no\" objFlags=\"00020001\" />\n\t\t\t\t\t</CANopenObject>\n\t\t\t\t\t<CANopenObject index=\"3002\" name=\"Auto start program\" objectType=\"7\" dataType=\"0005\" lowLimit=\"0\" highLimit=\"8\" accessType=\"rw\" defaultValue=\"0\" PDOmapping=\"no\" />\n\t\t\t\t\t<CANopenObject index=\"3003\" name=\"Access key\" objectType=\"7\" dataType=\"0007\" lowLimit=\"0\" highLimit=\"4294967295\" accessType=\"wo\" defaultValue=\"0\" PDOmapping=\"no\" objFlags=\"00020001\" />\n\t\t\t\t\t<CANopenObject index=\"3004\" name=\"Debug user program\" objectType=\"9\" subNumber=\"3\">\n\t\t\t\t\t\t<CANopenSubObject subIndex=\"00\" name=\"Number of entries\" objectType=\"7\" dataType=\"0005\" accessType=\"ro\" defaultValue=\"2\" PDOmapping=\"no\" />\n\t\t\t\t\t\t<CANopenSubObject subIndex=\"01\" name=\"Select variable\" objectType=\"7\" dataType=\"0005\" lowLimit=\"0\" highLimit=\"25\" accessType=\"rw\" defaultValue=\"0\" PDOmapping=\"no\" objFlags=\"00020000\" />\n\t\t\t\t\t\t<CANopenSubObject subIndex=\"02\" name=\"Selected variable value\" objectType=\"7\" dataType=\"0004\" lowLimit=\"-2147483648\" highLimit=\"2147483647\" accessType=\"rw\" defaultValue=\"0\" PDOmapping=\"no\" objFlags=\"00020000\" />\n\t\t\t\t\t</CANopenObject>\n\t\t\t\t\t<CANopenObject index=\"3005\" name=\"User program variables\" objectType=\"9\" subNumber=\"27\">\n\t\t\t\t\t\t<CANopenSubObject subIndex=\"00\" name=\"Number of entries\" objectType=\"7\" dataType=\"0005\" accessType=\"ro\" defaultValue=\"26\" PDOmapping=\"no\" />\n\t\t\t\t\t\t<CANopenSubObject subIndex=\"01\" name=\"User prog variable a\" objectType=\"7\" dataType=\"0004\" lowLimit=\"-2147483648\" highLimit=\"2147483647\" accessType=\"rw\" defaultValue=\"0\" PDOmapping=\"optional\" objFlags=\"00020001\" />\n\t\t\t\t\t\t<CANopenSubObject subIndex=\"02\" name=\"User prog variable b\" objectType=\"7\" dataType=\"0004\" lowLimit=\"-2147483648\" highLimit=\"2147483647\" accessType=\"rw\" defaultValue=\"0\" PDOmapping=\"optional\" objFlags=\"00020001\" />\n\t\t\t\t\t\t<CANopenSubObject subIndex=\"03\" name=\"User prog variable c\" objectType=\"7\" dataType=\"0004\" lowLimit=\"-2147483648\" highLimit=\"2147483647\" accessType=\"rw\" defaultValue=\"0\" PDOmapping=\"optional\" objFlags=\"00020001\" />\n\t\t\t\t\t\t<CANopenSubObject subIndex=\"04\" name=\"User prog variable d\" objectType=\"7\" dataType=\"0004\" lowLimit=\"-2147483648\" highLimit=\"2147483647\" accessType=\"rw\" defaultValue=\"0\" PDOmapping=\"optional\" objFlags=\"00020001\" />\n\t\t\t\t\t\t<CANopenSubObject subIndex=\"05\" name=\"User prog variable e\" objectType=\"7\" dataType=\"0004\" lowLimit=\"-2147483648\" highLimit=\"2147483647\" accessType=\"rw\" defaultValue=\"0\" PDOmapping=\"optional\" objFlags=\"00020001\" />\n\t\t\t\t\t\t<CANopenSubObject subIndex=\"06\" name=\"User prog variable f\" objectType=\"7\" dataType=\"0004\" lowLimit=\"-2147483648\" highLimit=\"2147483647\" accessType=\"rw\" defaultValue=\"0\" PDOmapping=\"optional\" objFlags=\"00020001\" />\n\t\t\t\t\t\t<CANopenSubObject subIndex=\"07\" name=\"User prog variable g\" objectType=\"7\" dataType=\"0004\" lowLimit=\"-2147483648\" highLimit=\"2147483647\" accessType=\"rw\" defaultValue=\"0\" PDOmapping=\"optional\" objFlags=\"00020001\" />\n\t\t\t\t\t\t<CANopenSubObject subIndex=\"08\" name=\"User prog variable h\" objectType=\"7\" dataType=\"0004\" lowLimit=\"-2147483648\" highLimit=\"2147483647\" accessType=\"rw\" defaultValue=\"0\" PDOmapping=\"optional\" objFlags=\"00020001\" />\n\t\t\t\t\t\t<CANopenSubObject subIndex=\"09\" name=\"User prog variable i\" objectType=\"7\" dataType=\"0004\" lowLimit=\"-2147483648\" highLimit=\"2147483647\" accessType=\"rw\" defaultValue=\"0\" PDOmapping=\"optional\" objFlags=\"00020001\" />\n\t\t\t\t\t\t<CANopenSubObject subIndex=\"0A\" name=\"User prog variable j\" objectType=\"7\" dataType=\"0004\" lowLimit=\"-2147483648\" highLimit=\"2147483647\" accessType=\"rw\" defaultValue=\"0\" PDOmapping=\"optional\" objFlags=\"00020001\" />\n\t\t\t\t\t\t<CANopenSubObject subIndex=\"0B\" name=\"User prog variable k\" objectType=\"7\" dataType=\"0004\" lowLimit=\"-2147483648\" highLimit=\"2147483647\" accessType=\"rw\" defaultValue=\"0\" PDOmapping=\"optional\" objFlags=\"00020001\" />\n\t\t\t\t\t\t<CANopenSubObject subIndex=\"0C\" name=\"User prog variable l\" objectType=\"7\" dataType=\"0004\" lowLimit=\"-2147483648\" highLimit=\"2147483647\" accessType=\"rw\" defaultValue=\"0\" PDOmapping=\"optional\" objFlags=\"00020001\" />\n\t\t\t\t\t\t<CANopenSubObject subIndex=\"0D\" name=\"User prog variable m\" objectType=\"7\" dataType=\"0004\" lowLimit=\"-2147483648\" highLimit=\"2147483647\" accessType=\"rw\" defaultValue=\"0\" PDOmapping=\"optional\" objFlags=\"00020001\" />\n\t\t\t\t\t\t<CANopenSubObject subIndex=\"0E\" name=\"User prog variable n\" objectType=\"7\" dataType=\"0004\" lowLimit=\"-2147483648\" highLimit=\"2147483647\" accessType=\"rw\" defaultValue=\"0\" PDOmapping=\"optional\" objFlags=\"00020001\" />\n\t\t\t\t\t\t<CANopenSubObject subIndex=\"0F\" name=\"User prog variable o\" objectType=\"7\" dataType=\"0004\" lowLimit=\"-2147483648\" highLimit=\"2147483647\" accessType=\"rw\" defaultValue=\"0\" PDOmapping=\"optional\" objFlags=\"00020001\" />\n\t\t\t\t\t\t<CANopenSubObject subIndex=\"10\" name=\"User prog variable p\" objectType=\"7\" dataType=\"0004\" lowLimit=\"-2147483648\" highLimit=\"2147483647\" accessType=\"rw\" defaultValue=\"0\" PDOmapping=\"optional\" objFlags=\"00020001\" />\n\t\t\t\t\t\t<CANopenSubObject subIndex=\"11\" name=\"User prog variable q\" objectType=\"7\" dataType=\"0004\" lowLimit=\"-2147483648\" highLimit=\"2147483647\" accessType=\"rw\" defaultValue=\"0\" PDOmapping=\"optional\" objFlags=\"00020001\" />\n\t\t\t\t\t\t<CANopenSubObject subIndex=\"12\" name=\"User prog variable r\" objectType=\"7\" dataType=\"0004\" lowLimit=\"-2147483648\" highLimit=\"2147483647\" accessType=\"rw\" defaultValue=\"0\" PDOmapping=\"optional\" objFlags=\"00020001\" />\n\t\t\t\t\t\t<CANopenSubObject subIndex=\"13\" name=\"User prog variable s\" objectType=\"7\" dataType=\"0004\" lowLimit=\"-2147483648\" highLimit=\"2147483647\" accessType=\"rw\" defaultValue=\"0\" PDOmapping=\"optional\" objFlags=\"00020001\" />\n\t\t\t\t\t\t<CANopenSubObject subIndex=\"14\" name=\"User prog variable t\" objectType=\"7\" dataType=\"0004\" lowLimit=\"-2147483648\" highLimit=\"2147483647\" accessType=\"rw\" defaultValue=\"0\" PDOmapping=\"optional\" objFlags=\"00020001\" />\n\t\t\t\t\t\t<CANopenSubObject subIndex=\"15\" name=\"User prog variable u\" objectType=\"7\" dataType=\"0004\" lowLimit=\"-2147483648\" highLimit=\"2147483647\" accessType=\"rw\" defaultValue=\"0\" PDOmapping=\"optional\" objFlags=\"00020001\" />\n\t\t\t\t\t\t<CANopenSubObject subIndex=\"16\" name=\"User prog variable v\" objectType=\"7\" dataType=\"0004\" lowLimit=\"-2147483648\" highLimit=\"2147483647\" accessType=\"rw\" defaultValue=\"0\" PDOmapping=\"optional\" objFlags=\"00020001\" />\n\t\t\t\t\t\t<CANopenSubObject subIndex=\"17\" name=\"User prog variable w\" objectType=\"7\" dataType=\"0004\" lowLimit=\"-2147483648\" highLimit=\"2147483647\" accessType=\"rw\" defaultValue=\"0\" PDOmapping=\"optional\" objFlags=\"00020001\" />\n\t\t\t\t\t\t<CANopenSubObject subIndex=\"18\" name=\"User prog variable x\" objectType=\"7\" dataType=\"0004\" lowLimit=\"-2147483648\" highLimit=\"2147483647\" accessType=\"rw\" defaultValue=\"0\" PDOmapping=\"optional\" objFlags=\"00020001\" />\n\t\t\t\t\t\t<CANopenSubObject subIndex=\"19\" name=\"User prog variable y\" objectType=\"7\" dataType=\"0004\" lowLimit=\"-2147483648\" highLimit=\"2147483647\" accessType=\"rw\" defaultValue=\"0\" PDOmapping=\"optional\" objFlags=\"00020001\" />\n\t\t\t\t\t\t<CANopenSubObject subIndex=\"1A\" name=\"User prog variable z\" objectType=\"7\" dataType=\"0004\" lowLimit=\"-2147483648\" highLimit=\"2147483647\" accessType=\"rw\" defaultValue=\"0\" PDOmapping=\"optional\" objFlags=\"00020001\" />\n\t\t\t\t\t</CANopenObject>\n\t\t\t\t\t<CANopenObject index=\"3006\" name=\"Scripting stack / Number of levels\" objectType=\"8\" subNumber=\"16\">\n\t\t\t\t\t\t<CANopenSubObject subIndex=\"00\" name=\"Number of levels\" objectType=\"7\" dataType=\"0005\" accessType=\"ro\" defaultValue=\"15\" PDOmapping=\"no\" objFlags=\"0001\" />\n\t\t\t\t\t\t<CANopenSubObject subIndex=\"01\" name=\"Call stack level 0\" objectType=\"7\" dataType=\"0006\" accessType=\"ro\" defaultValue=\"0x0\" PD
